vi "Check for Existing Insets.vi"(8 "error in":errorcluster, 11 "Inset in":refnum<class "Inset.lvclass">) -> (0 "error out":errorcluster, 3 "Inset out":refnum<class "Inset.lvclass">)   [LabVIEW 2019, in "Inset.lvclass"]
uses:
  Inset.lvclass
  Parse/Image/SVGImage.lvclass
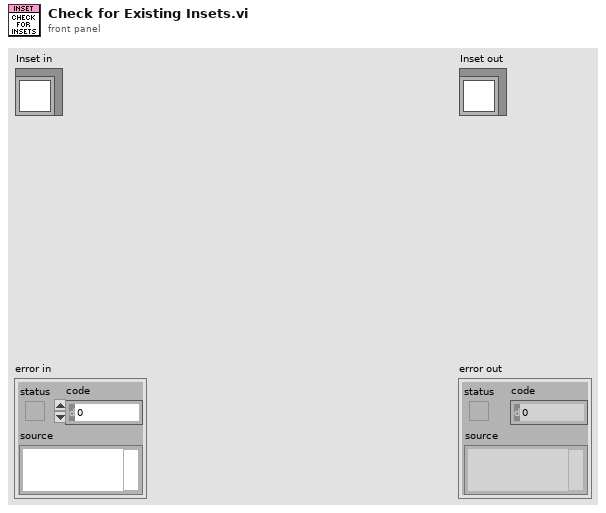
[diagram p1: front panel]
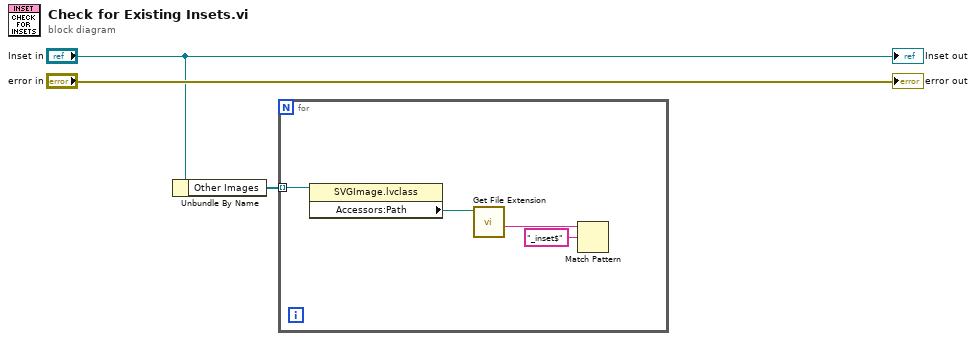
[diagram p0: block diagram]
diagram:
  n1 = Unbundle By Name("Inset in") -> ("Other Images"=w1:refnum<class "SVGImage.lvclass">[])
  n2 = for {
    tunnel: w1 -> [w7] mode=indexing
    n3 = property class="SVGImage.lvclass"(reference=w7) -> ("Accessors:Path"=w6:path)  [unwired: 1 in, 2 out]
    n4 = call <vilib>:"Get File Extension.vi"("file"=w6) -> ("filename without extension"=w5:string)  [unwired: 6 in, 4 out]
    n5 = Match Pattern(string=w5, regular expression="_inset$") -> ()  [unwired: 1 in, 4 out]
  }
  "error out" <- "error in"
  "Inset out" <- "Inset in"
